vi "SE_HV500.GetVoltage.vi"(0 "i ref in":refnum<vi>, 3 "Time out":i32, 5 "error in (no error)":errorcluster) -> (14 "i ref out":refnum<vi>, 16 "Read Voltage{V}":dbl format="%.2f", 17 "timed out":bool, 19 "error out":errorcluster)   [LabVIEW 2014]
doc: "Reads the Voltage in Volts at the output"
uses:
  SE_HV500.lvlib
  CSCore/CSSystem/CoreDefs/CoreDefs.error_type.ctl
  CSCore/CSSystem/CoreLib/CoreLib.lvlib
  CSlibraries-extern/DimLVEvent/LVDimInterface/LVDimInterface.lvlib
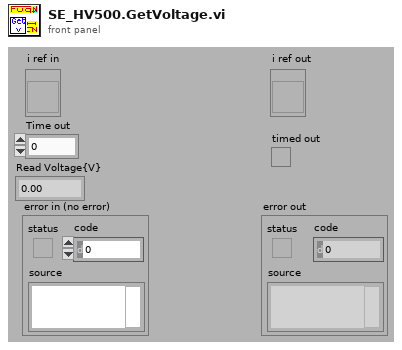
[diagram p1: front panel]
types:
  T1 = cluster{"VISA resource name":refnum<visa-resource-name>, "Gen time out":dbl, "timeout (0)":u32}
  T2 = typedef "CoreDefs.error_type.ctl" = enum16{"no error", "can't load process", "can't unload process", "process does not exist", "can't install process", "can't remove process", "unknown function", "time out", "can't execute function", "duplicate queue name", "super not found", "caller queue invalid", "can't ping process", "unknown error", "VISA Error", "VISA timeout", "GPIB timeout", "GPIB error", "communication error", "data type mismatch", "can't read data from OPC server", "can't write data to OPC server", "OET error", "function not implemented", "process already exists", "invalid Shared Variable name", "error writing Shared Variable", "error reading Shared Variable", "invalid client name", "corrupt database", "unknown class", "call not authorized", "parameter out of range", "OET timeout: can't get data to modify", "invalid queue name", "requested operation incompatible with current state", "event undefined", "event disabled", "state undefined", "caller is not a friend", "EventBuilder: bad eventID", "EventBuilder: no DAQ devices", "a thread must not stop itself", "UNUSED ELEMENT4", "DiscArchiver: eventData incomplete", "DiscArchiver: eventData does not belong to run", "DiscArchiver: can't open file", "DiscArchiver: can't write to file", "DiscArchiver: available disc space low", "can't acquire semaphore", "error reading data from database", "notifier object is not existing", "can't register process", "can't unregister process", "illegal event type", "object disabled", "object already exists", "can't change state", "Instrument not found", "no connection to remote node", "invalid reference", "N/A", "UNUSED ELEMENT 1", "element not found", "illegal TCP/IP connection detected", "object does not exist", "invalid access ID", "unknown CS system", "invalid privilige", "unsupported data type", "unsupported server type", "IO server already exists", "Shared Variable already exists"}
  T3 = typedef "SE_HV500.lvlib/SE_HV500.i attribute.ctl" = cluster{"SetStatus":bool, "Set Voltage":dbl, "VoltageID":i32, "Nom Voltage":dbl, "VISA resource name in":refnum<visa-resource-name>, "Device name":string, "PSRange":i32}
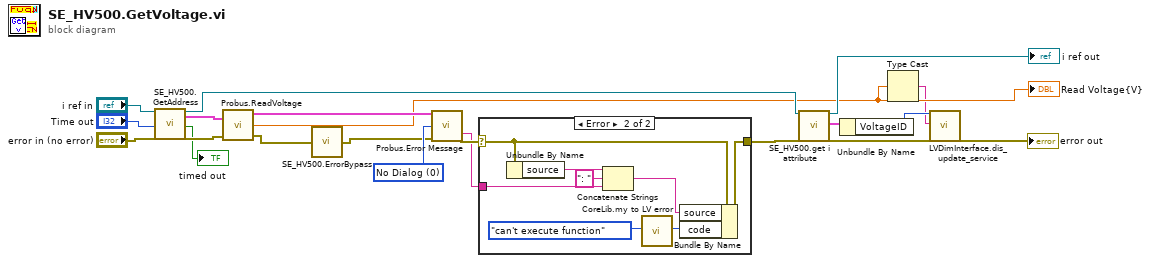
[diagram p0: block diagram]
diagram:
  w13 = 0 items=["No Dialog", "OK Message", "Continue or Stop Message"] ("Type of Dialog (1: OK Msg)")
  n1 = call "SE_HV500.GetAddress.vi"("i ref in"="i ref in", "Timeout"="Time out", "error in (no error)"="error in (no error)") -> ("i ref out"=w8:refnum<vi>, "VISA cluster out"=w19:T1, "timed out"=→"timed out":bool, "error out"=w18:errorcluster)  [unwired: 13 in]
  n2 = call "Probus.ReadVoltage.vi"("error in (no error)"=w18, "VISA cluster in"=w19) -> ("error out"=w2:errorcluster, "Read Voltage {V}"=w4:dbl, "VISA cluster out"=w15:T1)  [unwired: 1 in]
  "Read Voltage{V}" <- w4
  n3 = call "SE_HV500.ErrorBypass.vi"("error in (no error)"=w2) -> ("error out"=w1:errorcluster)  [unwired: 14 in]
  n4 = call "Probus.Error Message.vi"("Visa Cluster in"=w15, "Type of Dialog (1: OK Msg)"=w13, "error in (no error)"=w1) -> ("Error Message (empty)"=w12:string, "error out"=w14:errorcluster)  [unwired: 8 in, 3 out]
  n5 = case shown="Error" w14 {
    selector: w14 -> [w22 w27]
    tunnel: [w22 w29] -> w9
    tunnel: w12 -> [_ w24]
    frame No Error {
    }
    frame Error {
      n6 = Unbundle By Name(w27) -> ("source"=w26:string)
      n7 = Concatenate Strings(w26, ": " ("string"), w24) -> (w23:string)
      n8 = call "CoreLib.my to LV error.vi"("ErrorTypes"=CoreDefs.error_type."can't execute function") -> ("LV error code"=w28:i32)  [unwired: 17 in, 1 out]
      n9 = Bundle By Name(cluster=w27, "source"=w23, "code"=w28) -> (w29:errorcluster)
    }
  }
  n10 = call "SE_HV500.get i attribute.vi"("i ref in"=w8, "error in (no error)"=w9) -> ("i ref out"=→"i ref out":refnum<vi>, "i attribute"=w6:T3, "error out"=w10:errorcluster)  [unwired: 15 in]
  n11 = Unbundle By Name(w6) -> ("VoltageID"=w5:i32)
  n12 = Type Cast(x=w4) -> (*(type *) &x=w3:string)  [unwired: 1 in]
  n13 = call "LVDimInterface.dis_update_service.vi"("my_serviceID"=w5, "data"=w3, "error in (no error)"=w10) -> ("error out"=→"error out":errorcluster)  [unwired: 14 in, 2 out]
